vi "Get Results Metadata.vi"(7 "error in (no error)":errorcluster, 10 "MeasurementPluginService in":refnum<class "MeasurementPluginService.lvclass">) -> (0 "error out":errorcluster, 2 "Metadata Value":T2(array[cluster]), 3 "MeasurementPluginService out":refnum<class "MeasurementPluginService.lvclass">)   [LabVIEW 2020, in "MeasurementLink Measurement Server.lvlib"]
uses:
  MeasurementLink Measurement Server.lvlib
  TypeDefs/ConfigurationParameter_AnnotationsEntry.ctl
  Classes/MeasurementPluginService/MeasurementPluginService.lvclass
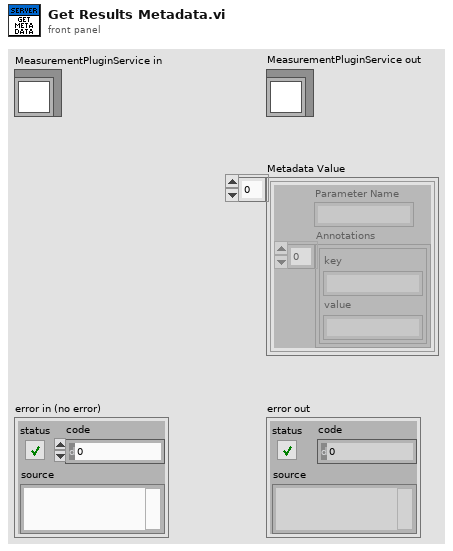
[diagram p1: front panel]
types:
  T1 = typedef "MeasurementLink Measurement Server.lvlib/ConfigurationParameter_AnnotationsEntry.ctl" = cluster{"key":string, "value":string}
  T2 = cluster{"Parameter Name":string, "Annotations":T1[]}[]
  T3 = typedef "MeasurementLink Measurement Server.lvlib/Parameter Type Specialization.ctl" = cluster{"Parameter Name":string, "Type Specialization":T4, "Annotations":cluster{"Key":T5, "Value":string}[]}
  T4 = typedef "MeasurementLink Measurement Server.lvlib/Type Specialization.ctl" = enum16{"none", "pin", "path", "enum"}
  T5 = typedef "MeasurementLink Measurement Server.lvlib/Type Specialization Key.ctl" = enum16{"none", "pin.instrument_type", "enum.values"}
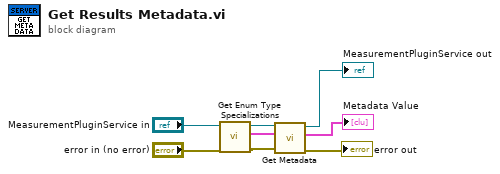
[diagram p0: block diagram]
diagram:
  n1 = call "Get Enum Type Specializations.vi"("error in (no error)"="error in (no error)", "MeasurementPluginService in"="MeasurementPluginService in") -> ("error out"=w6:errorcluster, "Type Specializations"=w4:T3[], "MeasurementPluginService out"=w3:refnum<class "MeasurementPluginService.lvclass">)  [unwired: 7 in]
  n2 = call "Get Metadata.vi"("error in (no error)"=w6, "Type Specializations"=w4, "MeasurementPluginService in"=w3) -> ("error out"=→"error out":errorcluster, "Metadata Value"=→"Metadata Value":T2, "MeasurementPluginService out"=→"MeasurementPluginService out":refnum<class "MeasurementPluginService.lvclass">)  [unwired: 5 in]
